vi "Set Grid (SubVI).vi"(5 "y offset":dbl, 7 "x offset":dbl, 8 "error in (no error)":errorcluster, 9 "index (row)":i32, 10 "ItemNames":string[][](array[string]), 11 "Application in":refnum<vi>) -> (0 "error out":errorcluster, 3 "Application out":refnum<vi>)   [LabVIEW 2014]
uses:
  <userlib>/Nanonis Prog Interface V5/Scan/Grid/GridPatternSet.vi
  <userlib>/Nanonis Prog Interface V5/Nanonis Prog Interface.lvlib
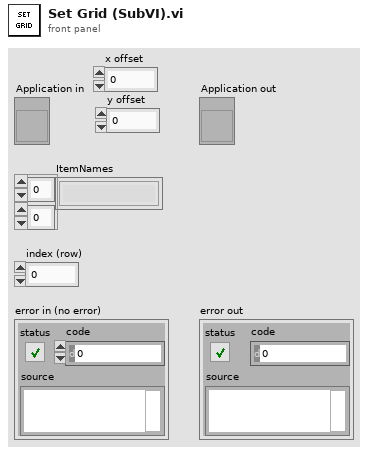
[diagram p1: front panel]
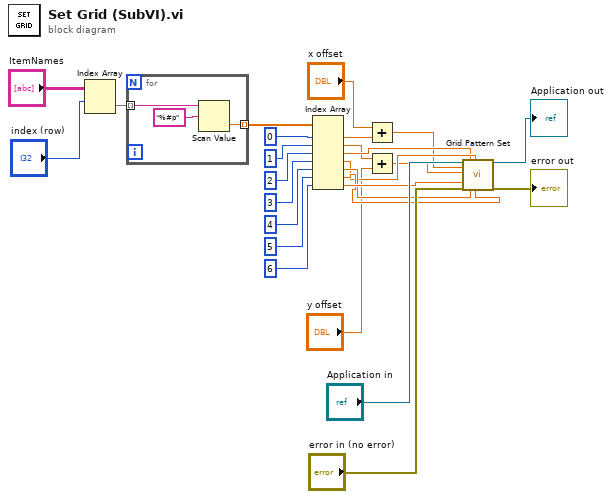
[diagram p0: block diagram]
diagram:
  n1 = Index Array(array="ItemNames", index (row)="index (row)") -> (element=w7:string[])  [unwired: 1 in]
  n2 = for {
    tunnel: w7 -> [w28] mode=indexing
    tunnel: [w27] -> w8 mode=indexing
    n3 = Scan Value(string=w28, format string="%#p") -> (value=w27:dbl)  [unwired: 1 in, 1 out]
  }
  n4 = Index Array(array=w8, index #1=0 ("index"), index #2=1 ("index"), index #3=2 ("index"), index #4=3 ("index"), index #5=4 ("index"), index #6=5 ("index"), index #7=6 ("index")) -> (element #1=w16:dbl, element #2=w17:dbl, element #3=w18:dbl, element #4=w19:dbl, element #5=w20:dbl, element #6=w21:dbl, element #7=w22:dbl)
  n5 = Add(x="x offset", y=w16) -> (x+y=w4:dbl)
  n6 = Add(x=w17, y="y offset") -> (x+y=w3:dbl)
  n7 = call-poly <userlib>:"Grid Pattern Set.vi"("Application ref in"="Application in", "Center Xc (m)"=w4, "Center Yc (m)"=w3, "Angle (°)"=w22, "error in (no error)"="error in (no error)", "Width (m)"=w18, "Points X"=w20, "Height (m)"=w19, "Points Y"=w21) -> ("Application ref out"=→"Application out":refnum<vi>, "error out"=→"error out":errorcluster)  [unwired: 9 in]
